vi "ImgPtrArrToImage.vi"(9 "CameraIndex":dbl, 11 "Image Pixels (U32)":u32[][](array[numeric])) -> (1 "error out":errorcluster, 3 "image out":T1(plugin-control))   [LabVIEW 2017, in "PlayNitrideCameraComponet1010_4.lvlib"]
uses:
  <userlib>/PlayNitrideCameraComponet1010_4/PlayNitrideCameraComponet1010_4.lvlib
panel:
  out "String":string
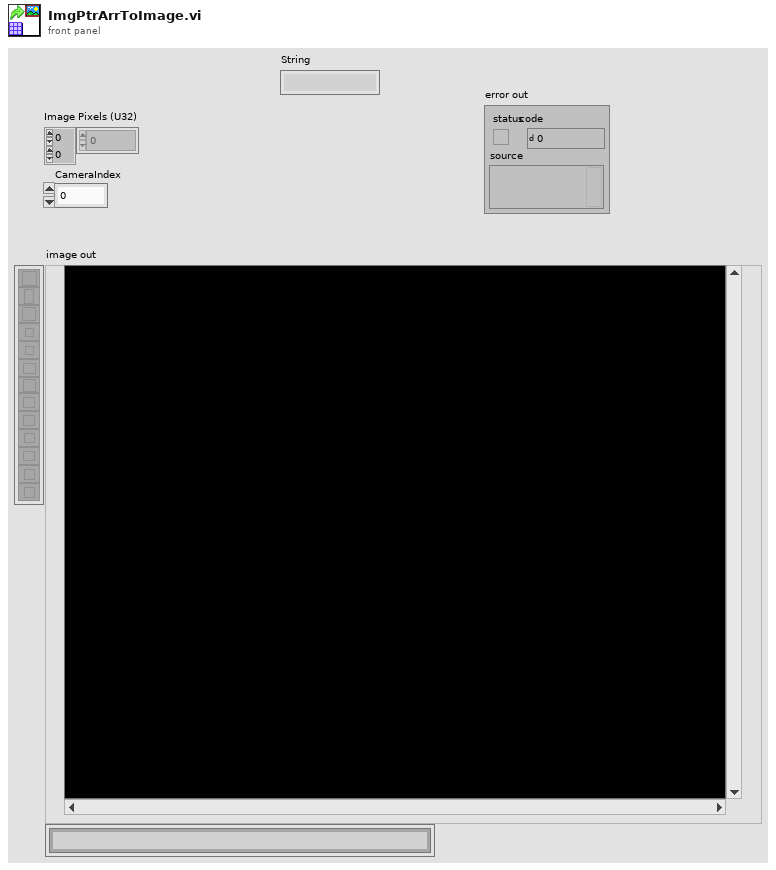
[diagram p1: front panel]
types:
  T1 = typedef "IMAQ Image.ctl" = refnum<image>
  T2 = typedef "Image Type" = u32
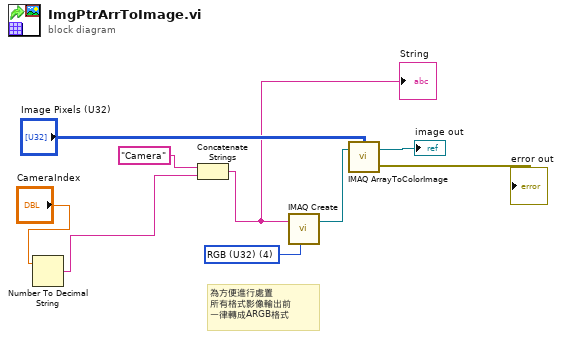
[diagram p0: block diagram]
diagram:
  w1 = T2 4 items=["Grayscale (U8)", "Grayscale (I16)", "Grayscale (SGL)", "Complex (CSG)", "RGB (U32)", "HSL (U32)", "RGB (U64)", "Grayscale (U16)"] ("Image Type")
  # "為方便進行處置\n所有格式影像輸出前\n一律轉成ARGB格式"
  n1 = Number To Decimal String(number="CameraIndex") -> (decimal integer string=w7:string)  [unwired: 1 in]
  n2 = Concatenate Strings("Camera" ("string"), w7) -> (w3:string)
  "String" <- w3
  n3 = call "IMAQ Create"("Image Name"=w3, "Image Type"=w1) -> ("New Image"=w5:T1)  [unwired: 3 in, 1 out]
  n4 = call "IMAQ ArrayToColorImage"("Image Pixels (U32)"="Image Pixels (U32)", "Image"=w5) -> ("Image Out"=→"image out":T1, "error out"=→"error out":errorcluster)  [unwired: 3 in]
